vi "Set-Image-height.vi"(8 "error in (no error)":errorcluster, 10 "Image height in":i32, 11 "PF_MV1-D1312-240 in":refnum<class "PF_MV1-D1312-240.lvclass">) -> (0 "error out":errorcluster, 1 "Image height delta":i32, 2 "Image height":i32, 3 "PF_MV1-D1312-240 out":refnum<class "PF_MV1-D1312-240.lvclass">)   [LabVIEW 2013, in "CameraVision.lvlib" / "PF_MV1-D1312-240.lvclass"]
uses:
  PF_MV1-D1312-240.lvclass
  Camera.lvclass/Camera.ctl
  <userlib>/Photonfocus Toolkit/_Public/SubVIs/pf_Set_Camera_Property_Int.vi
  <userlib>/Photonfocus Toolkit/Photonfocus_Toolkit.lvlib
  Camera.lvclass
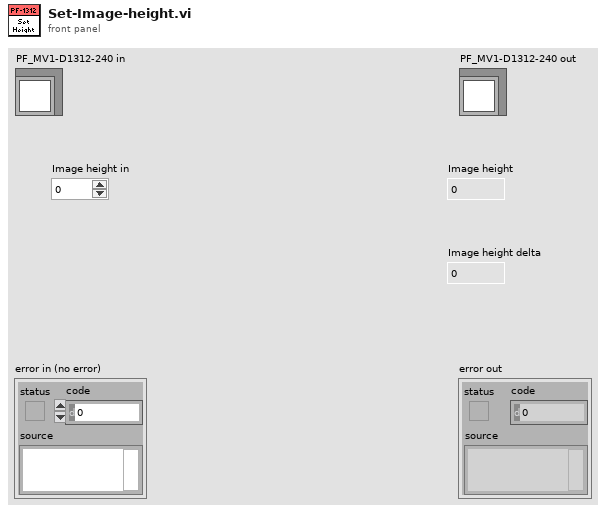
[diagram p1: front panel]
types:
  T1 = cluster{"Max. width":i32, "Max. height":i32, "Step size width":dbl, "Min. width":i32, "Min. height":i32, "Step size height":dbl}
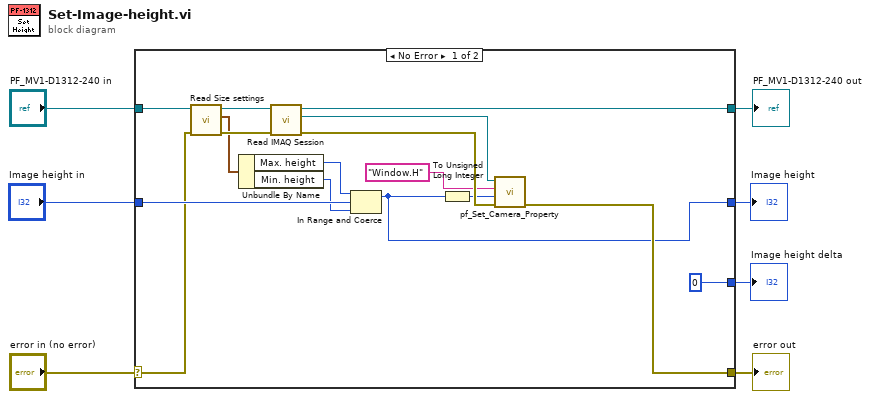
[diagram p0: block diagram]
diagram:
  n1 = case shown="No Error" "error in (no error)" {
    selector: "error in (no error)" -> [w14 w26]
    tunnel: [w20 w26] -> w6
    tunnel: [w22 w25] -> w4
    tunnel: "PF_MV1-D1312-240 in" -> [w12 w25]
    tunnel: "Image height in" -> [w18 w24]
    tunnel: [w17 w24] -> w2
    tunnel: [0 _] -> w1
    frame No Error {
      n2 = call-dynamic "Read Size settings.vi"("error in (no error)"=w14, "Camera in"=w12) -> ("error out"=w13:errorcluster, "Image size"=w10:T1, "Camera out"=w11:refnum<class "PF_MV1-D1312-240.lvclass">)  [unwired: 7 in]
      n3 = Unbundle By Name(w10) -> ("Max. height"=w8:i32, "Min. height"=w9:i32)
      n4 = call "Read IMAQ Session.vi"("error in (no error)"=w13, "Camera in"=w11) -> ("error out"=w21:errorcluster, "IMAQ Session"=w23:refnum<k11>, "Camera out"=w22:refnum<class "PF_MV1-D1312-240.lvclass">)  [unwired: 7 in]
      n5 = In Range and Coerce(upper limit=w8, x=w18, lower limit=w9) -> (coerced(x)=w17:i32)  [unwired: 1 out]
      n6 = To Unsigned Long Integer(number=w17) -> (unsigned 32bit integer=w15:u32)
      n7 = call-poly <userlib>:"pf_Set_Camera_Property.vi"("error in (no error)"=w21, "Property Value"=w15, "Property Name"="Window.H", "IMAQ Session in"=w23) -> ("error out"=w20:errorcluster)  [unwired: 5 in, 2 out]
    }
    frame Error {
    }
  }
  "error out" <- w6
  "PF_MV1-D1312-240 out" <- w4
  "Image height" <- w2
  "Image height delta" <- w1
